vi "Test Criteria, Record Result.vi"(6 "row (0)":u32, 8 "error in":errorcluster, 10 "Result":dbl format="%.3g", 11 "Tbl Refnum":refnum<vi>) -> (0 "error out":errorcluster, 3 "Tbl Refnum out":refnum<vi>, 4 "next row":u32)   [LabVIEW 2010]
doc: "This function records results in a Test Criteria table and marks them pass or fail."
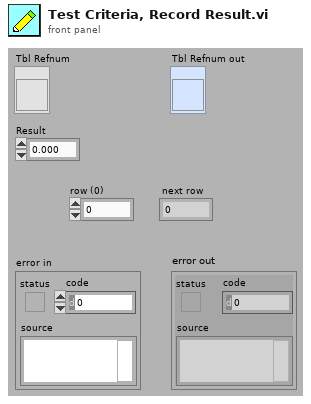
[diagram p1: front panel]
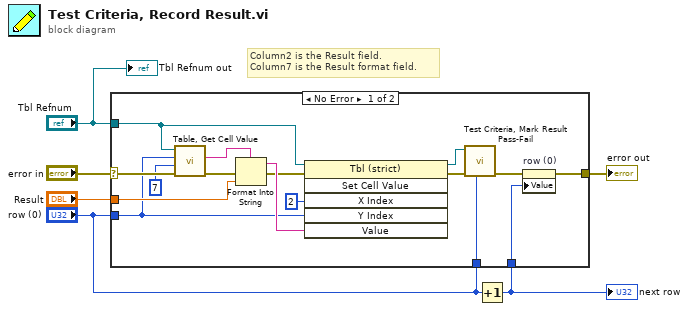
[diagram p0: block diagram]
diagram:
  # "Column2 is the Result field.\nColumn7 is the Result format field."
  n1 = Increment(x="row (0)") -> (x+1=w2:u32)
  "next row" <- w2
  n2 = case shown="No Error" "error in" {
    selector: "error in" -> [w18 w23]
    tunnel: [w9 w23] -> w6
    tunnel: "Tbl Refnum" -> [w12 _]
    tunnel: "row (0)" -> [w15 _]
    tunnel: "Result" -> [w20 _]
    tunnel: w2 -> [w13 _]
    tunnel: "row (0)" -> [w8 _]
    frame No Error {
      n3 = call "Table, Get Cell Value.vi"("error in"=w18, "column (0)"=u32 7 ("col_n"), "row (0)"=w15, "Tbl Refnum"=w12) -> ("error out"=w17:errorcluster, "cell value"=w16:string)  [unwired: 5 in, 1 out]
      n4 = Format Into String(format string=w16, error in=w17, w20) -> (resulting string=w21:string, error out=w19:errorcluster)  [unwired: 1 in]
      n5 = invoke class="Tbl (strict)" method="Set Cell Value"(reference=w12, error in=w19, "X Index"=u32 2, "Y Index"=w15, "Value"=w21) -> (reference out=w7:refnum<vi>, error out=w11:errorcluster)  [unwired: 1 in, 4 out]
      n6 = call "Test Criteria, Mark Result Pass-Fail.vi"("row (0)"=w8, "error in"=w11, "Tbl Refnum"=w7) -> ("error out"=w10:errorcluster)  [unwired: 7 in, 1 out]
      n7 = property on="row (0)" class="DigNum (strict)"(error in=w10, "Value"=w13) -> (error out=w9:errorcluster)  [unwired: 1 in, 1 out]
    }
    frame Error {
    }
  }
  "error out" <- w6
  "Tbl Refnum out" <- "Tbl Refnum"
